vi "Read.vi"(7 "error in (no error)":errorcluster, 9 "Frame Count":u32, 10 "SPI Ref In":T1={"myRIO Reference"={"myRIO Model"=enum."Unknown", "myRIO Hardware Reference"={"Generic FPGA Reference"=refnum, "Allow multiple opens"=FALSE}}, "SPI Channels Enum"=enum."Not Connected", "SPI Configuration"={"Frequency [Hz]"=0.0, "Clock Phase"=enum."Leading", "Clock Polarity"=enum."Low", "Data Direction"=enum."Most significant bit first", "Frame Length"=8}} {"SPI Configuration"."Frame Length" min=1 max=16}) -> (0 "error out":errorcluster, 1 "Frames Read":u16[](array[numeric]), 3 "SPI Ref Out":T1={"myRIO Reference"={"myRIO Model"=enum."Unknown", "myRIO Hardware Reference"={"Generic FPGA Reference"=refnum, "Allow multiple opens"=FALSE}}, "SPI Channels Enum"=enum."Not Connected", "SPI Configuration"={"Frequency [Hz]"=0.0, "Clock Phase"=enum."Leading", "Clock Polarity"=enum."Low", "Data Direction"=enum."Most significant bit first", "Frame Length"=8}} {"SPI Configuration"."Frame Length" min=1 max=16})   [LabVIEW 2021, in "SPI.lvlib"]
doc: "Reads a specified number of frames from a serial peripheral interface (SPI) channel. This VI returns results when all the frames are read. You use the Configure VI to specify the length of a frame."
uses:
  <vilib>/myRIO/Instrument Drivers/Onboard IO/SPI/SPI.lvlib
  <vilib>/myRIO/Instrument Drivers/Onboard IO/SPI/typedefs/SPI Reference.ctl
  <vilib>/myRIO/Common/Instrument Driver Framework/Utilities/typedefs/myRIO Generic Hardware Reference.ctl
  <vilib>/myRIO/Common/Instrument Driver Framework/Utilities/typedefs/Hardware Version Enum.ctl
  <vilib>/myRIO/Common/Instrument Driver Framework/Utilities/typedefs/myRIO v1.0 Reference.ctl
  <vilib>/myRIO/Common/Instrument Driver Framework/Utilities/typedefs/Generic FPGA Reference.ctl
  <vilib>/myRIO/Common/Instrument Driver Framework/myRIO v1.0/SPI/typedefs/SPI Channels Enum.ctl
  <vilib>/myRIO/Instrument Drivers/Onboard IO/SPI/typedefs/SPI Configuration.ctl
  <vilib>/myRIO/Common/Instrument Driver Framework/myRIO v1.0/SPI/typedefs/SPI Clock Phase.ctl
  <vilib>/myRIO/Common/Instrument Driver Framework/myRIO v1.0/SPI/typedefs/SPI Clock Polarity.ctl
  <vilib>/myRIO/Common/Instrument Driver Framework/myRIO v1.0/SPI/typedefs/SPI Data Direction.ctl
  <vilib>/myRIO/Common/Instrument Driver Framework/myRIO v1.0/SPI/typedefs/SPI Frame Length.ctl
  <vilib>/myRIO/Common/Instrument Driver Framework/myRIO v1.0/SPI/vis/myRIO v1.0 Write Read SPI.vi
  <vilib>/myRIO/Common/Instrument Driver Framework/ELVIS III v1.0/SPI/vis/ELVIS III v1.0 Write Read SPI.vi
  <vilib>/myRIO/Common/Instrument Driver Framework/roboRIO v1.0/SPI/vis/roboRIO v1.0 Write Read SPI.vi
  <vilib>/Utility/error.llb/Error Cluster From Error Code.vi
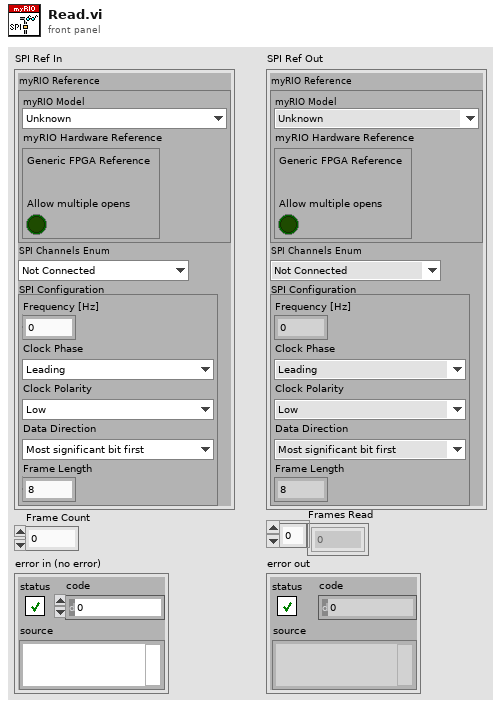
[diagram p1: front panel]
types:
  T1 = typedef "SPI.lvlib/SPI Reference.ctl" = cluster{"myRIO Reference":T2, "SPI Channels Enum":T6, "SPI Configuration":T7}
  T2 = typedef "myRIO Generic Hardware Reference.ctl" = cluster{"myRIO Model":T3, "myRIO Hardware Reference":T4}
  T3 = typedef "Hardware Version Enum.ctl" = enum16{"Unknown", "myRIO-1900", "myRIO-1950", "roboRIO", "NI ELVIS RIO CM", "ELVIS III"}
  T4 = typedef "myRIO v1.0 Reference.ctl" = cluster{"Generic FPGA Reference":T5, "Allow multiple opens":bool}
  T5 = typedef "Generic FPGA Reference.ctl" = refnum<k20>
  T6 = typedef "SPI Channels Enum.ctl" = enum16{"Not Connected", "A/SPI", "B/SPI", "SPI/SPI"}
  T7 = typedef "SPI.lvlib/SPI Configuration.ctl" = cluster{"Frequency [Hz]":dbl, "Clock Phase":T8, "Clock Polarity":T9, "Data Direction":T10, "Frame Length":T11}
  T8 = typedef "SPI Clock Phase.ctl" = enum8{"Leading", "Trailing"}
  T9 = typedef "SPI Clock Polarity.ctl" = enum8{"Low", "High"}
  T10 = typedef "SPI Data Direction.ctl" = enum8{"Most significant bit first", "Least significant bit first"}
  T11 = typedef "SPI Frame Length.ctl" = u8
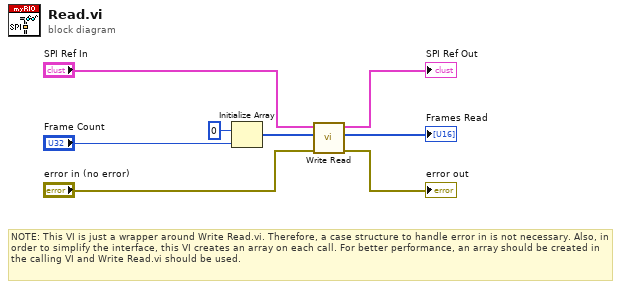
[diagram p0: block diagram]
diagram:
  # "NOTE: This VI is just a wrapper around Write Read.vi. Therefore, a case structure to handle error in is not necessary. Also, in order to simplify the interface, this VI creates an array on each call. For better performance, an array should be created in the calling VI and Write Read.vi should be used."
  n1 = Initialize Array(u16 0 ("element"), "Frame Count") -> (w1:u16[])
  n2 = call <vilib>:"Write Read.vi"("error in (no error)"="error in (no error)", "Frames to Write"=w1, "SPI Ref In"="SPI Ref In") -> ("error out"=→"error out":errorcluster, "Frames Read"=→"Frames Read":u16[], "SPI Ref Out"=→"SPI Ref Out":T1)  [unwired: 6 in]
